vi "Pockels Cal-Remove last row if empty strings.vi"(11 "Pockels Cal table":string[][](array[string])=[["Cal Wavelength", "", "", ""], ["820", "", "", ""], ["Prism 1:", "2039", "", ""], ["Prism 2:", "1953", "", ""], ["Laser power displayed (mW):", "3960", "", ""], ["Pockels bias:", "199", "", ""], ["Zoom:", "12", "", ""], ["Dwell time:", "0.4", "", ""], ["Cal subset indexes", "", "", ""], ["0", "15", "", ""], ["Cal data", "", "", ""], ["Pockels V", "No objective", "Nikon X", "Nikon 25X"], ["0", "0", "", "0"], ["0.1", "2.8", "", "1.96"], ["0.2", "9.8", "", "6.86"], ["0.3", "21.4", "", "14.98"], ["0.4", "37.1", "", "25.97"], ["0.5", "56.1", "", "39.27"], ["0.6", "77.7", "", "54.39"], ["0.7", "101", "", "70.7"], ["0.8", "125", "", "87.5"], ["0.9", "148", "", "103.6"], ["1", "169", "", "118.3"], ["1.1", "188", "", "131.6"], ["1.2", "204", "", "142.8"], ["1.3", "215", "", "150.5"], ["1.4", "222", "", "155.4"], ["1.5", "225", "", "157.5"], ["1.6", "222", "", "155.4"], ["1.7", "214", "", "149.8"], ["1.8", "202", "", "141.4"], ["1.9", "187", "", "130.9"], ["2", "152", "", "106.4"]]) -> (3 "Pockels Cal table (inc. header line)":string[][](array[string]))   [LabVIEW 2020]
panel:
  out "Last row removed (was empty strings)":bool
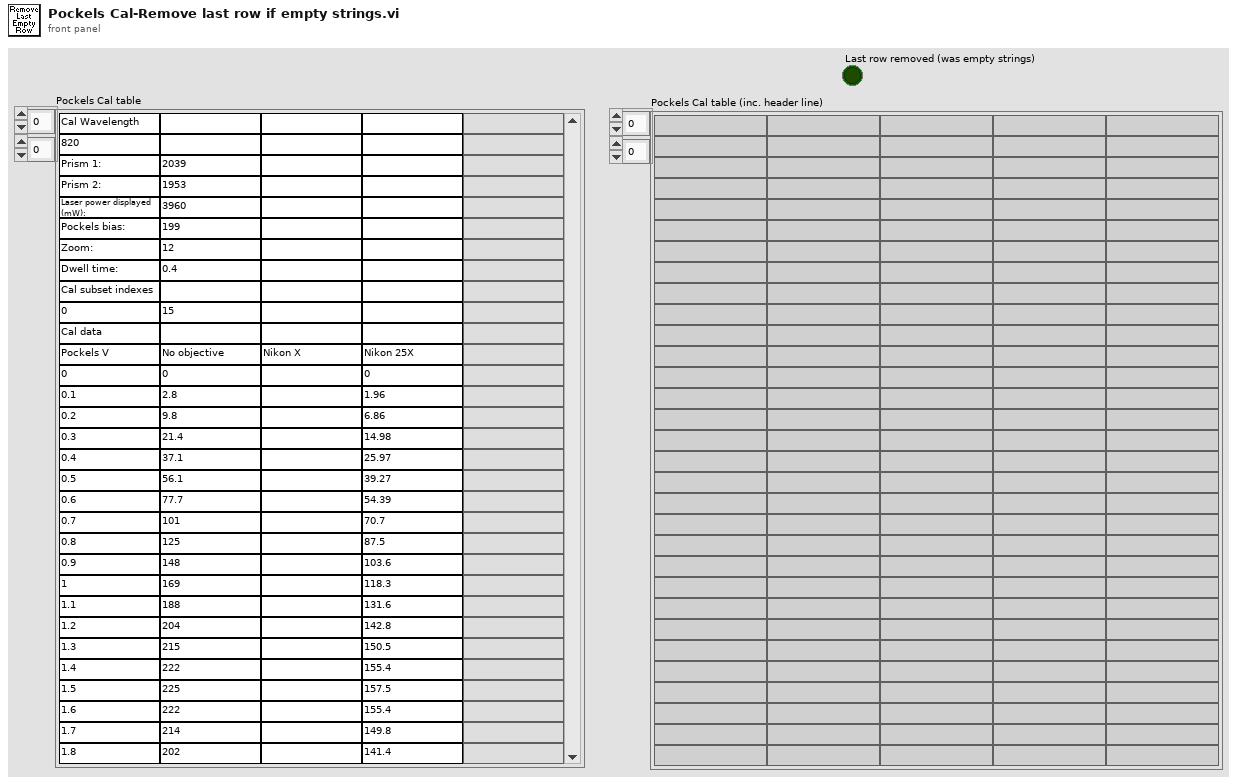
[diagram p1: front panel]
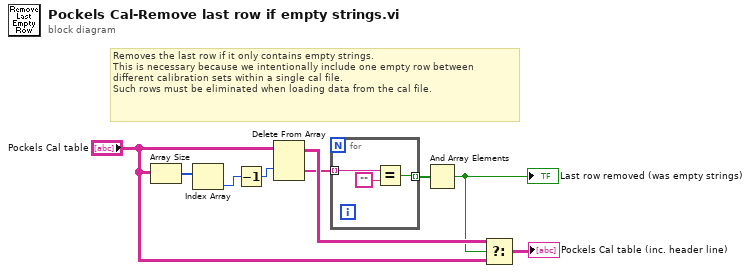
[diagram p0: block diagram]
diagram:
  # "Removes the last row if it only contains empty strings.\nThis is necessary because we intentionally include one empty row between different calibration sets within a single cal file.\nSuch rows must be eliminated when loading data from the cal file."
  n1 = Array Size(array="Pockels Cal table") -> (size(s)=w1:i32[])
  n2 = Index Array(array=w1) -> (element=w2:i32)  [unwired: 1 in]
  n3 = Decrement(x=w2) -> (x-1=w3:i32)
  n4 = Delete From Array(array="Pockels Cal table", index (row)=w3) -> (deleted portion=w4:string[], array with subset deleted=w7:string[][])  [unwired: 2 in]
  n5 = for {
    tunnel: w4 -> [w12] mode=indexing
    tunnel: [w10] -> w5 mode=indexing
    n6 = Equal?(x=w12, y="") -> (x = y?=w10:bool)
  }
  n7 = And Array Elements(Boolean array=w5) -> (logical AND=w6:bool)
  "Last row removed (was empty strings)" <- w6
  n8 = Select(t=w7, s=w6, f="Pockels Cal table") -> (s? t:f=→"Pockels Cal table (inc. header line)":string[][])
